vi "Init.vi"(8 "error in (no error)":errorcluster caption="错误输入（无错误）", 10 "size":i32=128, 11 "FIFO(DBL) 输入":refnum<class "FIFO(U32).lvclass"> caption="DNL_LabVIEW Object in") -> (0 "error out":errorcluster caption="错误输出", 3 "FIFO(DBL) 输出":refnum<class "FIFO(U32).lvclass"> caption="DNL_LabVIEW Object out")   [LabVIEW 2012, in "FIFO(U32).lvclass"]
uses:
  FIFO(U32).lvclass
  FIFO(U32).lvclass/FIFO(U32).ctl
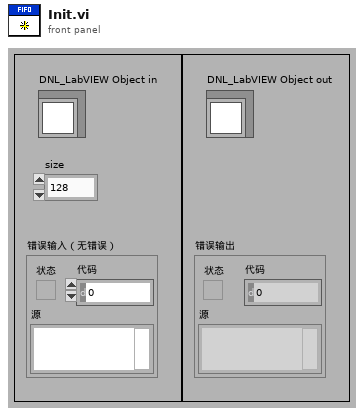
[diagram p1: front panel]
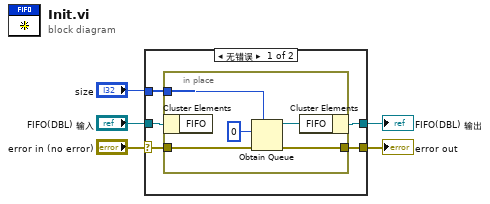
[diagram p0: block diagram]
diagram:
  n1 = case shown="无错误" "error in (no error)" {
    selector: "error in (no error)" -> [w9 w17]
    tunnel: [w8 w17] -> w4
    tunnel: [w7 w16] -> w2
    tunnel: "FIFO(DBL) 输入" -> [w10 w16]
    tunnel: "size" -> [w6 _]
    frame No Error {
      n2 = in-place {
        in-place-border: w9 -> [w15]
        in-place-border: [w14] -> w8
        in-place-border: w6 -> [w11]
        n3 = in-place-cluster #1(w10) -> ()  [unwired: 1 out]
        n4 = Obtain Queue(max queue size (-1, unlimited)=w11, element data type=u32 0, error in (no error)=w15) -> (queue out=w12:refnum<queue>, error out=w14:errorcluster)  [unwired: 2 in, 1 out]
        n5 = in-place-cluster #1("FIFO"=w12) -> (w7:refnum<class "FIFO(U32).lvclass">)
      }
    }
    frame Error {
    }
  }
  "error out" <- w4
  "FIFO(DBL) 输出" <- w2
